vi "CheesyDrive.vi"(6 "Quickturn":bool, 7 "SlowMode":u32, 8 "Fast Mode":bool, 10 "Wheel":dbl(slide)=-0.015748031496062992 scale=-1.0..1.0, 11 "Throttle":dbl(slide)=0.007874015748031496 scale=-1.0..1.0) -> (2 "Right PWM":dbl, 3 "Left PWM":dbl)   [LabVIEW 2019]
doc: "Implements CheesyDrive. CheesyDrive means that the turn joystick controls the radius of turning instead of the rate of turning. Also implements QuickStop and QuickTurn."
panel:
  in  "ArrayOfSlownesss":T1(array[cluster])=[{"MaxSpeedSlow"=1.0, "SlowRate"=5.0, "MaxTurnSlow"=1.0, "MaxTurnRateSlow"=8.0}, {"MaxSpeedSlow"=0.6, "SlowRate"=4.0, "MaxTurnSlow"=0.8, "MaxTurnRateSlow"=10.0}, {"MaxSpeedSlow"=0.4, "SlowRate"=3.0, "MaxTurnSlow"=0.75, "MaxTurnRateSlow"=10.0}]
  in  "PointsTurn":cluster{"X":dbl, "Y":dbl}[](array[cluster])=[{"X"=0.0, "Y"=0.0}, {"X"=0.04, "Y"=0.0}, {"X"=0.041, "Y"=0.01}, {"X"=0.6, "Y"=0.3}, {"X"=1.0, "Y"=1.0}]
  in  "PointsQuickTurn":cluster{"X":dbl, "Y":dbl}[](array[cluster])=[{"X"=0.0, "Y"=0.0}, {"X"=0.05, "Y"=0.05}, {"X"=1.0, "Y"=0.6}]
  in  "PointsThrottle":cluster{"X":dbl, "Y":dbl}[](array[cluster])=[{"X"=0.0, "Y"=0.0}, {"X"=0.025, "Y"=0.0}, {"X"=1.0, "Y"=0.75}]
  in  "QSMult":dbl=0.12
  in  "WheelNonLinearity":dbl=0.01
  in  "negInertiaScalar":dbl=4.0
  in  "alpha":dbl=0.1
  out "QuickStop Value":dbl(graph)
  in  "Sensitivty":dbl=1.0
  # "These are the inputs and outputs\nNot configuration"
  # "Check block diagram for details on these"
  # "normal"
  # "Switch"
  # "Scale"
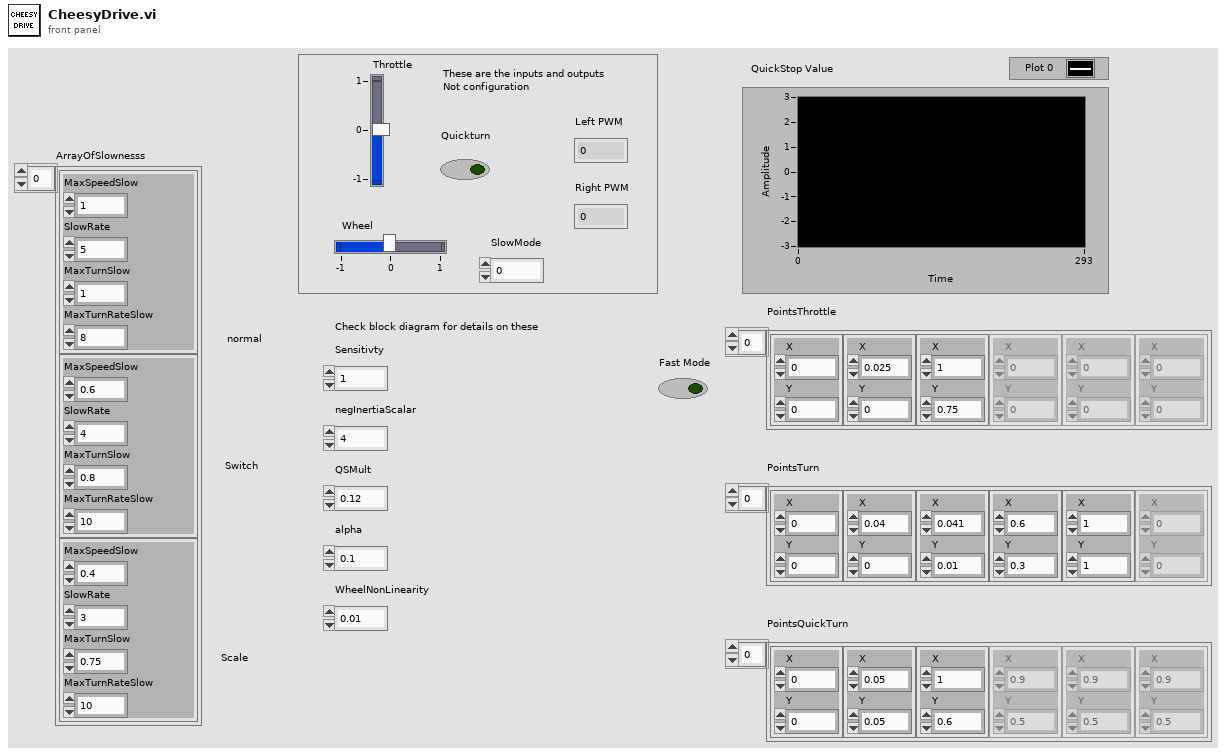
[diagram p1: front panel]
types:
  T1 = cluster{"MaxSpeedSlow":dbl, "SlowRate":dbl, "MaxTurnSlow":dbl, "MaxTurnRateSlow":dbl}[]
  T2 = cluster{"MaxSpeedSlow":dbl, "SlowRate":dbl, "MaxTurnSlow":dbl, "MaxTurnRateSlow":dbl}
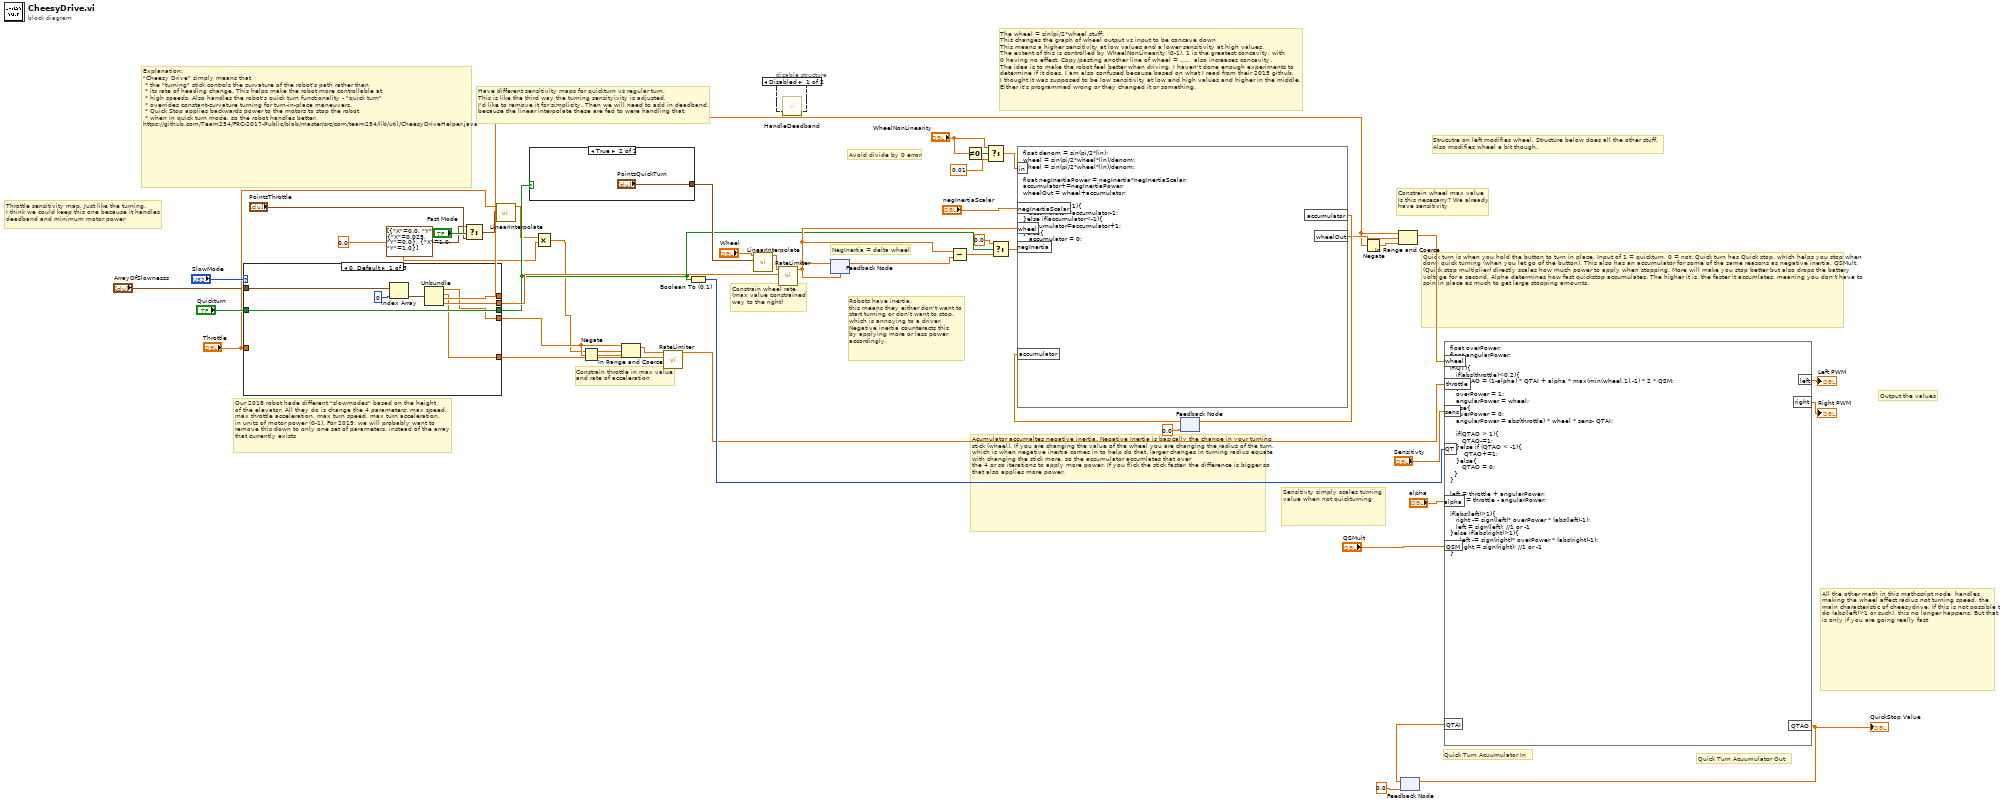
[diagram p0: block diagram]
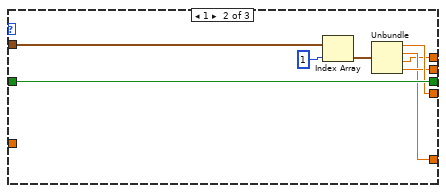
[diagram p3: hidden frame]
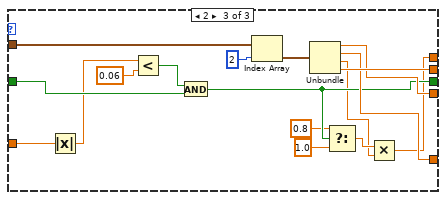
[diagram p4: hidden frame]
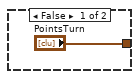
[diagram p5: hidden frame]
diagram:
  # "Strucutre on left modifies wheel. Structure below does all the other stuff.\nAlso modifies wheel a bit though."
  # "Sensitivty simply scales turning value when not quickturning"
  # "All the other math in this mathscript node  handles making the wheel affect radius not turning speed, the main characteristic of cheesydrive. If this is not possible to do (abs(left)>1 or such), this no longer happens. But that is only if you are going really fast"
  # "Quick turn is when you hold the button to turn in place. Input of 1 = quickturn, 0 = not. Quick turn has Quick stop, which helps you stop when done quick turning (when you let go of the button). This also has an accumulator for some of the same reasons as negative inertia. QSMult, (Quick stop multiplier) directly scales how much power to apply when stopping. More will make you stop better but also drops the battery voltage for a second. Alpha determines how fast quickstop accumulates. The higher it is, the faster it accumlates, meaning you don't have to spin in place as much to get large stopping amounts."
  # "Output the values"
  # "Acumulator accumaltes negative inertia. Negative Inertia is basically the change in your turning stick (wheel). If you are changing the value of the wheel you are changing the radius of the turn, which is when negative inertia comes in to help do that. larger changes in turning radius equate with changing the stick more, so the accumulator accumlates that over\nthe 4 or so iterations to apply more power. If you flick the stick faster, the difference is bigger so that also applies more power."
  # "The wheel = sin(pi/2*wheel stuff:\nThis changes the graph of wheel output vs input to be concave down\nThis means a higher sensitivity at low values and a lower sensitivity at high values.\nThe extent of this is controlled by WheelNonLinearity (0-1). 1 is the greatest concavity, with\n0 having no effect. Copy/pasting another line of wheel = .....  also increases concavity.\nThe idea is to make the robot feel better when driving. I haven't done enough experiments to \ndetermine if it does. I am also confused because based on what I read from their 2015 github,\nI thought it was supposed to be low sensitivity at low and high values and higher in the middle.\nEither it's programmed wrong or they changed it or something."
  # "Constrain wheel max value\nIs this necesarry? We already\nhave sensitivity"
  # "Constrain wheel rate\n(max value constrained\nway to the right)"
  # "Throttle sensitivity map. Just like the turning,\nI think we could keep this one because it handles\ndeadband and minimum motor power"
  # "Have different sensitivity maps for quickturn vs regular turn.\nThis is like the third way the turning sensityivity is adjusted. \nI'd like to remove it for simplicity. Then we will need to add in deadband,\nbecause the linear interpolate these are fed to were handling that."
  # "Robots have inertia.\nthis means they either don't want to\nstart turning or don't want to stop,\nwhich is annoying to a driver. \nNegative inertia counteracts this\nby applying more or less power\naccordingly."
  # "Constrain throttle in max value\nand rate of acceleration"
  # "Our 2018 robot hade different \"slowmodes\" based on the height\nof the elevator. All they do is change the 4 parameters: max speed,\nmax throttle acceleration, max turn speed, max turn acceleration,\nin units of motor power (0-1). For 2019, we will probably want to\nremove this down to only one set of parameters, instead of the array\nthat currently exists"
  # "Avoid divide by 0 error"
  # "NegInertia = delta wheel"
  # "Explanation:\n\"Cheesy Drive\" simply means that\n * the \"turning\" stick controls the curvature of the robot's path rather than\n * its rate of heading change. This helps make the robot more controllable at\n * high speeds. Also handles the robot's quick turn functionality - \"quick turn\"\n * overrides constant-curvature turning for turn-in-place maneuvers.\n * Quick Stop applies backwards power to the motors to stop the robot\n * when in quick turn mode, so the robot handles better.\nhttps://github.com/Team254/FRC-2017-Public/blob/master/src/com/team254/lib/util/CheesyDriveHelper.java"
  # "Quick Turn Acuumulator Out"
  # "Quick Turn Acuumulator In"
  n1 = case shown="0, Default" "SlowMode" {
    tunnel: [w48 w57 w71] -> w27
    tunnel: [w49 w59 w73] -> w12
    tunnel: [w50 w56 w64] -> w25
    tunnel: [w51 w58 w74] -> w23
    tunnel: "Quickturn" -> [w55 w63 w80]
    tunnel: [w55 w63 w68] -> w16
    tunnel: "Throttle" -> [_ _ w72]
    tunnel: "ArrayOfSlownesss" -> [w52 w60 w77]
    frame 0, Default {
      n2 = Index Array(array=w52, index=0) -> (element=w53:T2)
      n3 = Unbundle(w53) -> ("MaxSpeedSlow"=w49:dbl, "SlowRate"=w48:dbl, "MaxTurnSlow"=w50:dbl, "MaxTurnRateSlow"=w51:dbl)
    }
    frame 1 {
      n4 = Index Array(array=w60, index=1) -> (element=w61:T2)
      n5 = Unbundle(w61) -> ("MaxSpeedSlow"=w59:dbl, "SlowRate"=w57:dbl, "MaxTurnSlow"=w56:dbl, "MaxTurnRateSlow"=w58:dbl)
    }
    frame 2 {
      n6 = Absolute Value(x=w72) -> (abs(x)=w70:dbl)
      n7 = Less?(x=w70, y=0.06) -> (x < y?=w79:bool)
      n8 = And(x=w79, y=w80) -> (x .and. y?=w68:bool)
      n9 = Index Array(array=w77, index=2) -> (element=w75:T2)
      n10 = Unbundle(w75) -> ("MaxSpeedSlow"=w73:dbl, "SlowRate"=w71:dbl, "MaxTurnSlow"=w65:dbl, "MaxTurnRateSlow"=w74:dbl)
      n11 = Select(t=0.8, s=w68, f=1.0) -> (s? t:f=w66:dbl)
      n12 = Multiply(x=w66, y=w65) -> (x*y=w64:dbl)
    }
  }
  n13 = Select(t=cluster{"X":dbl, "Y":dbl}[] [{"X"=0.0, "Y"=0.0}, {"X"=0.025, "Y"=0.0}, {"X"=1.0, "Y"=1.0}] ("PointsThrottle"), s="Fast Mode", f="PointsThrottle") -> (s? t:f=w4:cluster{"X":dbl, "Y":dbl}[])
  n14 = call "LinearInterpolate.vi"("Points"=w4, "Value"="Throttle") -> ("Output"=w3:dbl)  [unwired: 9 in]
  n15 = case shown="True" w16 {
    tunnel: ["PointsTurn" "PointsQuickTurn"] -> w29
    frame False {
    }
    frame True {
    }
  }
  n16 = Multiply(x=w3, y=0.0) -> (x*y=w2:dbl)
  n17 = Negate(x=w12) -> (-x=w13:dbl)
  n18 = In Range and Coerce(upper limit=w12, x=w2, lower limit=w13) -> (coerced(x)=w14:dbl)  [unwired: 1 out]
  n19 = call "RateLimiter.vi"("Max dx/dt"=w27, "Input"=w14) -> ("Output"=w41:dbl)  [unwired: 9 in]
  n20 = Boolean To (0,1)(Boolean=w16) -> (0, 1=w45:i16)
  n21 = call "LinearInterpolate.vi"("Points"=w29, "Value"="Wheel") -> ("Output"=w24:dbl)  [unwired: 9 in]
  n22 = disable-structure shown="Disabled" {
    frame Disabled {
      n23 = call "HandleDeadband.vi"() -> ()  [unwired: 11 in, 1 out]
    }
    frame Enabled {
    }
  }
  n24 = call "RateLimiter.vi"("Max dx/dt"=w23, "Input"=w24) -> ("Output"=w30:dbl)  [unwired: 9 in]
  n25 = feedback #1(w30) -> (w38:dbl)
  n26 = feedback-in #1(w30) -> ()
  n27 = Subtract(x=w30, y=w38) -> (x-y=w21:dbl)
  n28 = Not Equal To 0?(x="WheelNonLinearity") -> (x != 0?=w11:bool)
  n29 = Select(t="WheelNonLinearity", s=w11, f=0.01) -> (s? t:f=w8:dbl)
  n30 = Select(t=0.0, s=w16, f=w21) -> (s? t:f=w22:dbl)
  n31 = feedback #2(0.0 ("Wheel")) -> (w37:dbl)
  n32 = formula code="float denom = sin(pi/2*lin);\nwheel = sin(pi/2*wheel*lin)/denom;\nwheel = sin(pi/2*wheel*lin)/denom;\n\nfloat negInertiaPower = negInertia*negInertiaScalar;\naccumulator+=negInertiaPower;\nwheelOut = wheel+accumulator;\n\nif(accumulator>1){\n   accumulator=accumulator-1;\n}else if(accumulator<-1){\n   accumulator=accumulator+1;\n}else{\n   accumulator = 0;\n}"("wheel"=w30, "negInertia"=w22, "accumulator"=w37, "negInertiaScalar"="negInertiaScalar", "lin"=w8) -> ("accumulator"=w35:dbl, "wheelOut"=w32:dbl)
  n33 = feedback-in #2(w35) -> ()
  n34 = Negate(x=w25) -> (-x=w26:dbl)
  n35 = In Range and Coerce(upper limit=w25, x=w32, lower limit=w26) -> (coerced(x)=w33:dbl)  [unwired: 1 out]
  n36 = feedback #3(0.0 ("QTAccumulatorO")) -> (w43:dbl)
  n37 = formula code="float overPower;\nfloat angularPower;\n\nif(QT){\n   if(abs(throttle)<0.2){\n      QTAO = (1-alpha) * QTAI + alpha * max(min(wheel,1),-1) * 2 * QSM;\n   }\n   overPower = 1;\n   angularPower = wheel;\n}else{\n   overPower = 0;\n   angularPower = abs(throttle) * wheel * sens- QTAI;\n\n   if(QTAO > 1){\n      QTAO-=1;\n   }else if (QTAO < -1){\n       QTAO+=1;\n   }else{\n      QTAO = 0;\n  }\n}\n\nleft = throttle + angularPower;\nright = throttle - angularPower;\n\nif(abs(left)>1){\n   right -= sign(left)* overPower * (abs(left)-1);\n   left = sign(left); //1 or -1\n}else if(abs(right)>1){\n     left -= sign(right)* overPower * (abs(right)-1);\n     right = sign(right); //1 or -1 \n}"("wheel"=w33, "throttle"=w41, "sens"="Sensitivty", "QT"=w45, "alpha"="alpha", "QTAI"=w43, "QSM"="QSMult") -> ("left"=→"Left PWM":dbl, "right"=→"Right PWM":dbl, "QTAO"=w46:dbl)
  "QuickStop Value" <- w46
  n38 = feedback-in #3(w46) -> ()
